vi "Camera_AveYUV.vi"(2 "SRV In":string) -> (1 "YUV":cluster{"Y":sgl, "U":sgl, "V":sgl}, 4 "SRV Out":string="169.254.0.10")   [LabVIEW 2009]
panel:
  out "data out":string
  # "This LabVIEW item is deprecated.\n\nIt is believed to be unused and will be removed in a future version of SRV."
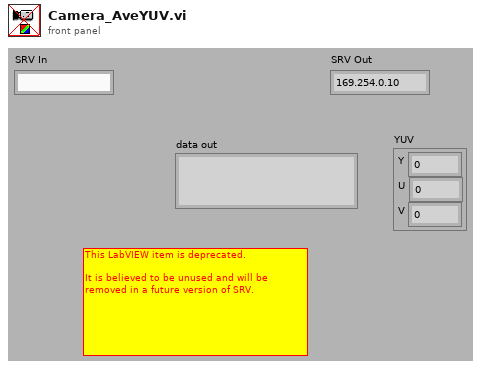
[diagram p1: front panel]
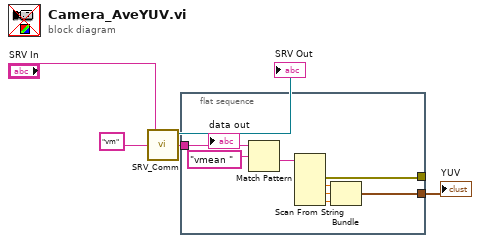
[diagram p0: block diagram]
diagram:
  n1 = call "SRV_Comm.vi"("Command Sent"="vm", "SRV In"="SRV In") -> ("Reply"=w5:string, "SRV Out"=→"SRV Out":refnum<k5>)  [unwired: 1 in, 1 out]
  n2 = flat-sequence {
    tunnel: w5 -> [w13]
    tunnel: [w10] -> _
    tunnel: [w6] -> w1
    frame #0 {
      n3 = Match Pattern(string=w13, regular expression="vmean " ("Command Sent")) -> (after substring=w12:string)  [unwired: 1 in, 3 out]
      n4 = Scan From String(input string=w12) -> (error out=w10:errorcluster, output 1=w7:dbl, output 2=w8:dbl, output 3=w9:dbl)  [unwired: 6 in, 2 out]
      n5 = Bundle(w7, w8, w9) -> (w6:cluster{dbl, dbl, dbl})  [unwired: 1 in]
      "data out" <- w13
    }
  }
  "YUV" <- w1
